vi "Usage Acceleration.vi"() -> ()   [LabVIEW 2011, in "Wiimote.lvlib"]
uses:
  Wiimote.lvlib
  Wiimote Buttons.ctl
panel:
  in  "index":i32
  out "Wiimote Buttons out":T1
  in  "stop":bool
  out "Waveform Chart":T2(graph)
  out "error out":errorcluster
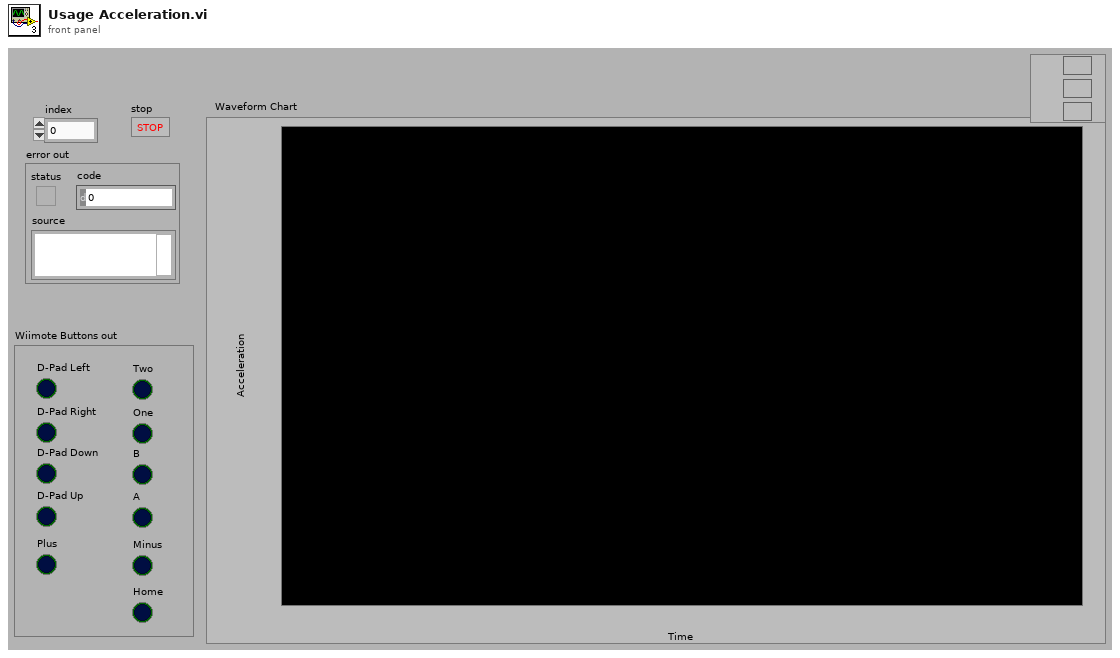
[diagram p1: front panel]
types:
  T1 = typedef "Wiimote.lvlib/Wiimote Buttons.ctl" = cluster{"D-Pad Left":bool, "D-Pad Right":bool, "D-Pad Down":bool, "D-Pad Up":bool, "Plus":bool, "Two":bool, "One":bool, "B":bool, "A":bool, "Minus":bool, "Home":bool}
  T2 = cluster{"Acceleration X":dbl, "Acceleration Y":dbl, "Acceleration Z":dbl}
  T3 = typedef "Wiimote.lvlib/Wiimote Acceleration.ctl" = cluster{"Acceleration X":dbl, "Acceleration Y":dbl, "Acceleration Z":dbl}
  T4 = cluster{"Wiimote 0G Calibration":T3, "Wiimote 1G Calibration":T3, "Nunchuk 0G Calibration":T3, "Nunchuk 1G Calibration":T3}
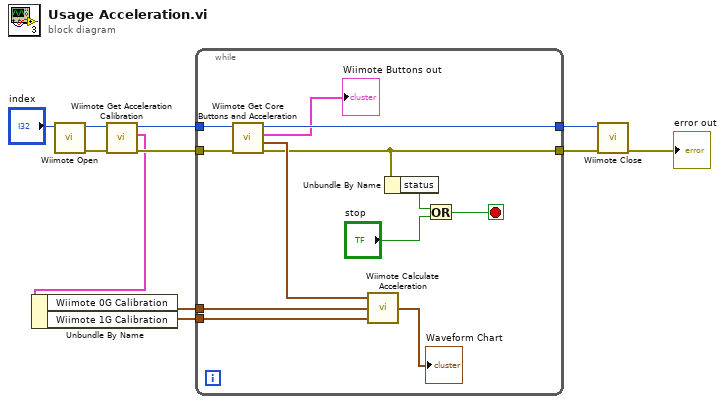
[diagram p0: block diagram]
diagram:
  n1 = call "Wiimote Open.vi"("index"="index") -> ("error out"=w5:errorcluster, "hWiimoteHandle"=w6:u32)  [unwired: 9 in]
  n2 = call "Wiimote Get Acceleration Calibration.vi"("error in"=w5, "hWiimoteHandle in"=w6) -> ("error out"=w7:errorcluster, "Calibration Data Out"=w3:T4, "hWiimoteHandle out"=w8:u32)  [unwired: 7 in]
  n3 = Unbundle By Name(w3) -> ("Wiimote 0G Calibration"=w2:T3, "Wiimote 1G Calibration"=w1:T3)
  n4 = while {
    tunnel: [w20] -> w10
    tunnel: [w23] -> w9
    tunnel: w8 -> [w16]
    tunnel: w7 -> [w15]
    tunnel: w2 -> [w13]
    tunnel: w1 -> [w12]
    stop <- w18 stop-if-true
    n5 = call "Wiimote Get Core Buttons and Acceleration.vi"("error in"=w15, "hWiimoteHandle in"=w16) -> ("error out"=w20:errorcluster, "Wiimote Acceleration out"=w22:T3, "Wiimote Buttons out"=→"Wiimote Buttons out":T1, "hWiimoteHandle out"=w23:u32)  [unwired: 6 in]
    n6 = call "Wiimote Calculate Acceleration.vi"("Acceleration 1G Calibration"=w12, "Acceleration 0G Calibration"=w13, "Acceleration Raw in"=w22) -> ("Acceleration Calibrated Out"=→"Waveform Chart":T3)
    n7 = Unbundle By Name(w20) -> ("status"=w19:bool)
    n8 = Or(x=w19, y="stop") -> (x .or. y?=w18:bool)
  }
  n9 = call "Wiimote Close.vi"("error in"=w10, "hWiimoteHandle in"=w9) -> ("error out"=→"error out":errorcluster)  [unwired: 9 in]
